vi "DSF.Engine.Execution.Plugin.Set ID.vi"(8 "error in (no error)":errorcluster, 10 "id":i32, 11 "Plugin in":refnum<class "DSF.Engine.Execution.Plugin.lvclass">) -> (0 "error out":errorcluster, 3 "Plugin out":refnum<class "DSF.Engine.Execution.Plugin.lvclass">)   [LabVIEW 2016, in "DSF.Engine.lvlib" / "DSF.Engine.Execution.Plugin.lvclass"]
uses:
  DSF.Engine.Execution.Plugin.lvclass
  DSF.Engine.Execution.Plugin.lvclass/DSF.Engine.Execution.Plugin.ctl
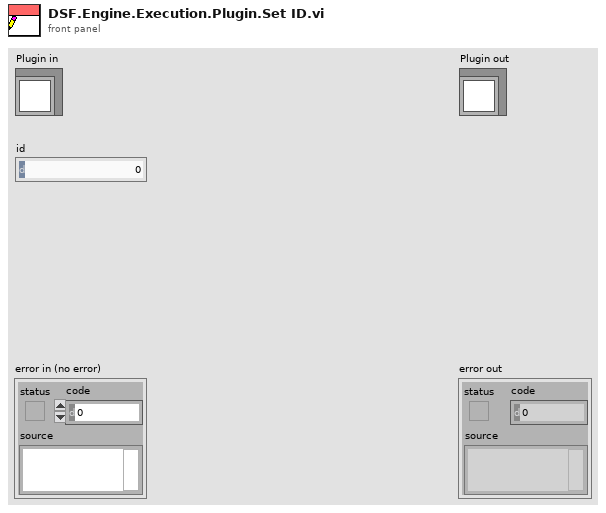
[diagram p1: front panel]
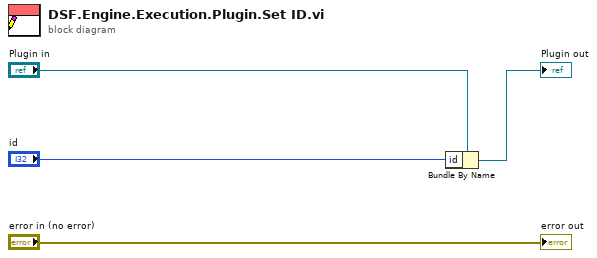
[diagram p0: block diagram]
diagram:
  n1 = Bundle By Name(cluster="Plugin in", "id"="id") -> (→"Plugin out":refnum<class "DSF.Engine.Execution.Plugin.lvclass">)
  "error out" <- "error in (no error)"
